vi "OC2 Send command.vi"(0 "VISA resource name":refnum<visa-resource-name>, 1 "Command data":string, 2 "Command":string, 3 "error in (no error)":errorcluster, 4 "coms":bool=TRUE) -> (5 "dup VISA resource name":refnum<visa-resource-name>, 6 "error out":errorcluster)   [LabVIEW 2023]
doc: "TCM Send command.vi\n\nLow level VI that sends data commands to the TCM\n\nCOPYRIGHT ELECTRON DYNAMICS LTD"
panel:
  out "unsigned byte array 2":u8[](array[numeric])
  out "return count":u32
  out "checksum":u8 format="%.0x"
  out "unsigned byte array":u8[](array[numeric])
  out "Data sent":string
  out "length":i32
  # "Send command"
  # "V1.02"
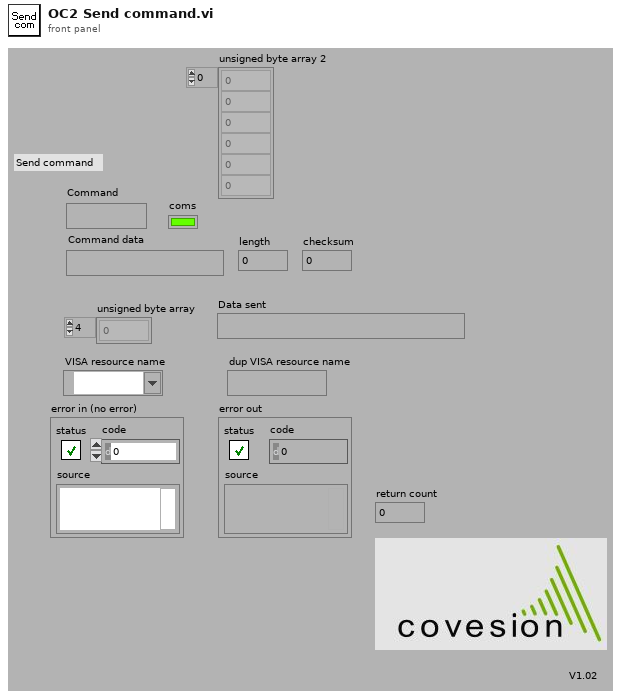
[diagram p1: front panel]
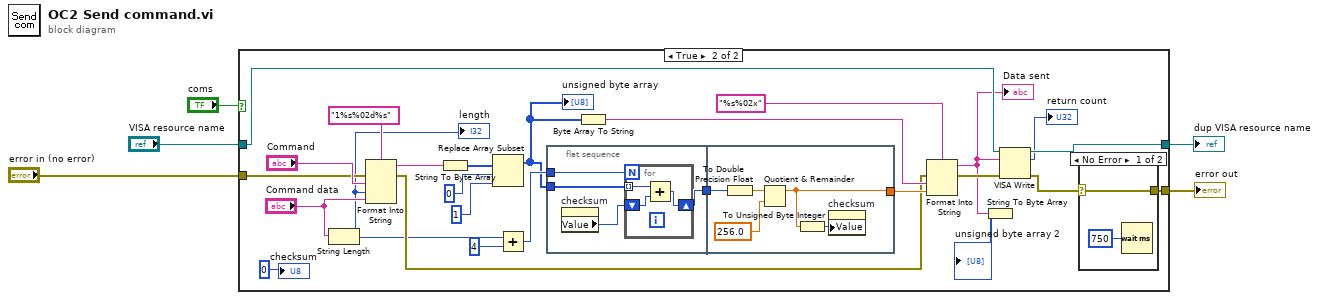
[diagram p0: block diagram]
diagram:
  n1 = case shown="True" "coms" {
    tunnel: "VISA resource name" -> [w7 w19]
    tunnel: [w7 w18] -> w4
    tunnel: [w6 w10] -> w1
    tunnel: "error in (no error)" -> [w6 w17]
    frame False {
    }
    frame True {
      n2 = String Length(string="Command data") -> (length=w13:i32)
      "length" <- w13
      n3 = Format Into String(format string="1%s%02d%s", error in=w17, "Command", w13, "Command data") -> (resulting string=w22:string, error out=w15:errorcluster)  [unwired: 1 in]
      n4 = String To Byte Array(string=w22) -> (unsigned byte array=w21:u8[])
      n5 = Replace Array Subset(array=w21, new element=u8 1, index=0) -> (w20:u8[])
      "unsigned byte array" <- w20
      n6 = Add(x=w13, y=4) -> (x+y=w28:i32)
      n7 = flat-sequence {
        tunnel: w28 -> [w39]
        tunnel: w20 -> [w40]
        tunnel: [w38] -> w12
        tunnel: [w45] -> w23
        tunnel: w12 -> [w47]
        frame #0 {
          n8 = property on="checksum" class="DigNum (strict)"() -> ("Value"=w37:u8)  [unwired: 2 in, 2 out]
          n9 = for {
            N: w39 -> [_]
            tunnel: w40 -> [w43] mode=indexing
            shift-right: [w42] -> w38
            shift-left: w37 -> [w41]
            n10 = Add(x=w43, y=w41) -> (x+y=w42:u8)
          }
        }
        frame #1 {
          n11 = To Double Precision Float(number=w47) -> (double precision float=w46:dbl)
          n12 = Quotient & Remainder(x=w46, y=256.0) -> (x-y*floor(x/y)=w45:dbl)  [unwired: 1 out]
          n13 = To Unsigned Byte Integer(number=w45) -> (unsigned 8bit integer=w44:u8)
          n14 = property on="checksum" class="DigNum (strict)"("Value"=w44) -> ()  [unwired: 2 in, 2 out]
        }
      }
      n15 = Byte Array To String(unsigned byte array=w20) -> (string=w24:string)
      n16 = Format Into String(format string="%s%02x", error in=w15, w24, w23) -> (resulting string=w9:string, error out=w14:errorcluster)  [unwired: 1 in]
      "Data sent" <- w9
      n17 = String To Byte Array(string=w9) -> (unsigned byte array=→"unsigned byte array 2":u8[])
      n18 = VISA Write(VISA resource name=w19, write buffer=w9, error in (no error)=w14) -> (VISA resource name out=w18:refnum<visa-resource-name>, return count=→"return count":u32, error out=w11:errorcluster)
      n19 = case shown="No Error" w11 {
        selector: w11 -> [w35 w36]
        tunnel: [w35 w36] -> w10
        frame No Error {
          n20 = Wait (ms)(milliseconds to wait=u32 750) -> ()  [unwired: 1 out]
        }
        frame Error {
        }
      }
      "checksum" <- 0 ("checksum")
    }
  }
  "dup VISA resource name" <- w4
  "error out" <- w1
